vi "Global allarme combinazione DO.vi"() -> ()   [LabVIEW 2019]
panel:
  out "Allarme combinazione DO":bool
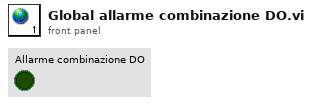
[diagram p1: front panel]
diagram:
